vi "Test1.vi"() -> ()   [LabVIEW 2012]
uses:
  <vilib>/Rock Robotics/SystemInterfaces/DIO/FPGA_DIOPWMChannel.ctl
  <vilib>/Rock Robotics/SystemInterfaces/Typedef/FPGA_TypedefDigitalModule.ctl
  <vilib>/Rock Robotics/SystemInterfaces/DIO/FPGA_DIOChannel.ctl
  <vilib>/Rock Robotics/WPI/Encoder/WPI_EncoderType.ctl
  <vilib>/Rock Robotics/WPI/MotorControl/WPI_MotorControlOpen Talon.vi
  <vilib>/Rock Robotics/WPI/Counter/WPI_CounterDigitalInputToDigitalSource.vi
  <vilib>/addons/control/pid/pid.llb/PID (DBL).vi
  <vilib>/addons/control/pid/NI_PID_pid.lvlib
panel:
  out "Numeric":dbl
  in  "stop":bool
  out "Times run":i32
  out "Ready To Fire":bool
  in  "Shooter Speed":dbl format="%.2f"
  in  "PID gains":T1={"proportional gain (Kc)"=1.0, "integral time (Ti, min)"=0.01, "derivative time (Td, min)"=0.0} {"derivative time (Td, min)" format="%.3f"; "integral time (Ti, min)" format="%.3f"; "proportional gain (Kc)" format="%.3f"}
  in  "Maximum Encoder speed":dbl=25000.0
  in  "Shooter On":bool
  # "This is the new code for the Shooter Motors. Check and make sure that all of the controls/indecators below work and that \nit exports the data to the dashboard correctly"
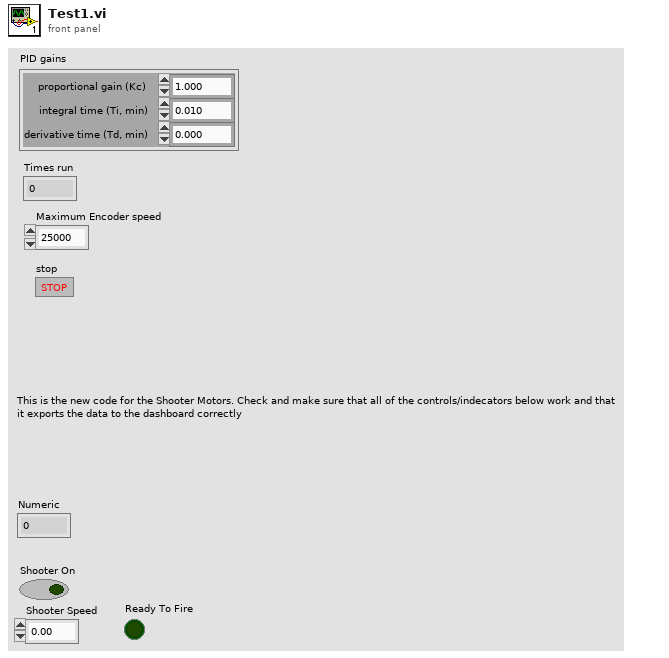
[diagram p1: front panel]
types:
  T1 = cluster{"proportional gain (Kc)":dbl, "integral time (Ti, min)":dbl, "derivative time (Td, min)":dbl}
  T2 = typedef "WPI_EncoderType.ctl" = enum16{"1x", "2x", "4x"}
  T3 = typedef "FPGA_DIOChannel.ctl" = enum8{"DIO 1", "DIO 2", "DIO 3", "DIO 4", "DIO 5", "DIO 6", "DIO 7", "DIO 8", "DIO 9", "DIO 10", "DIO 11", "DIO 12", "DIO 13", "DIO 14", "Invalid"}
  T4 = typedef "FPGA_DIOPWMChannel.ctl" = enum8{"PWM 1", "PWM 2", "PWM 3", "PWM 4", "PWM 5", "PWM 6", "PWM 7", "PWM 8", "PWM 9", "PWM 10", "Invalid"}
  T5 = typedef "FPGA_TypedefDigitalModule.ctl" = enum16{"Digital Module 1", "Digital Module 2"}
  T6 = typedef "WPI_DigitalInputDevRef.ctl" = cluster{"DevStatus":errorcluster, "DIO Channel":T3, "Digital Module":T5}
  T7 = typedef "FPGA_CounterEncoderSourceConvertionLVSourceType.ctl" = cluster{"DevStatus":errorcluster, "AnalogTriggerMode?":bool, "DigitalMode":cluster{"Digital Module":T5, "DIO Channel":T8}, "AnalogTriggerMode":cluster{"AnalogTriggerIndex":T9, "OutputType":T10}}
  T8 = typedef "FPGA_DIODigitalSourceChannel.ctl" = enum8{"DIO 1", "DIO 2", "DIO 3", "DIO 4", "DIO 5", "DIO 6", "DIO 7", "DIO 8", "DIO 9", "DIO 10", "DIO 11", "DIO 12", "DIO 13", "DIO 14", "Disabled"}
  T9 = typedef "FPGA_AnalogTriggerIndex.ctl" = enum8{"Trig 0", "Trig 1", "Trig 2", "Trig 3", "Trig 4", "Trig 5", "Trig 6", "Trig 7", "Invalid"}
  T10 = typedef "FPGA_AnalogTriggerOutType.ctl" = enum16{"InWindow", "TriggerState", "Rising", "Falling"}
  T11 = typedef "WPI_MotorControlDeviceRef.ctl" = cluster{"DeviceStatus":errorcluster, "Type":enum16{"PWM", "CAN"}, "PWM":cluster{"Digital Module":T5, "PWM Channel":T4, "DeadBand":T12}, "CAN":cluster{"Device Number":u8, "Control Mode":T13, "Semaphore":T14, "Max Vout":dbl}, "Invert":bool, "TransformRef":T15, "InvTransformRef":T15}
  T12 = typedef "WPI_PWMDeadband.ctl" = cluster{"Name":string, "maxPositivePwm":i32, "minPositivePwm":i32, "centerPwm":i32, "maxNegativePwm":i32, "minNegativePwm":i32, "angularRange":u16}
  T13 = typedef "WPI_CANJaguar_ControlMode.ctl" = enum8{"Percent VBus", "Current", "Speed", "Position", "Voltage"}
  T14 = typedef "Semaphore RefNum" = refnum<k1>
  T15 = typedef "WPI_PWMTransform_ConPane.ctl" = refnum<vi>
  T16 = typedef "WPI_EncoderDevRef.ctl" = cluster{"DevStatus":errorcluster, "EncoderIndex":T17, "CounterIndex":T18, "DistancePerCount":dbl, "Decoding Type":T2}
  T17 = typedef "FPGA_EncoderIdx.ctl" = enum8{"Enc 0", "Enc 1", "Enc 2", "Enc 3", "Invalid"}
  T18 = typedef "FPGA_CounterCtrSystemIndex.ctl" = enum8{"Ctr 0", "Ctr 1", "Ctr 2", "Ctr 3", "Ctr 4", "Ctr 5", "Ctr 6", "Ctr 7", "Invalid"}
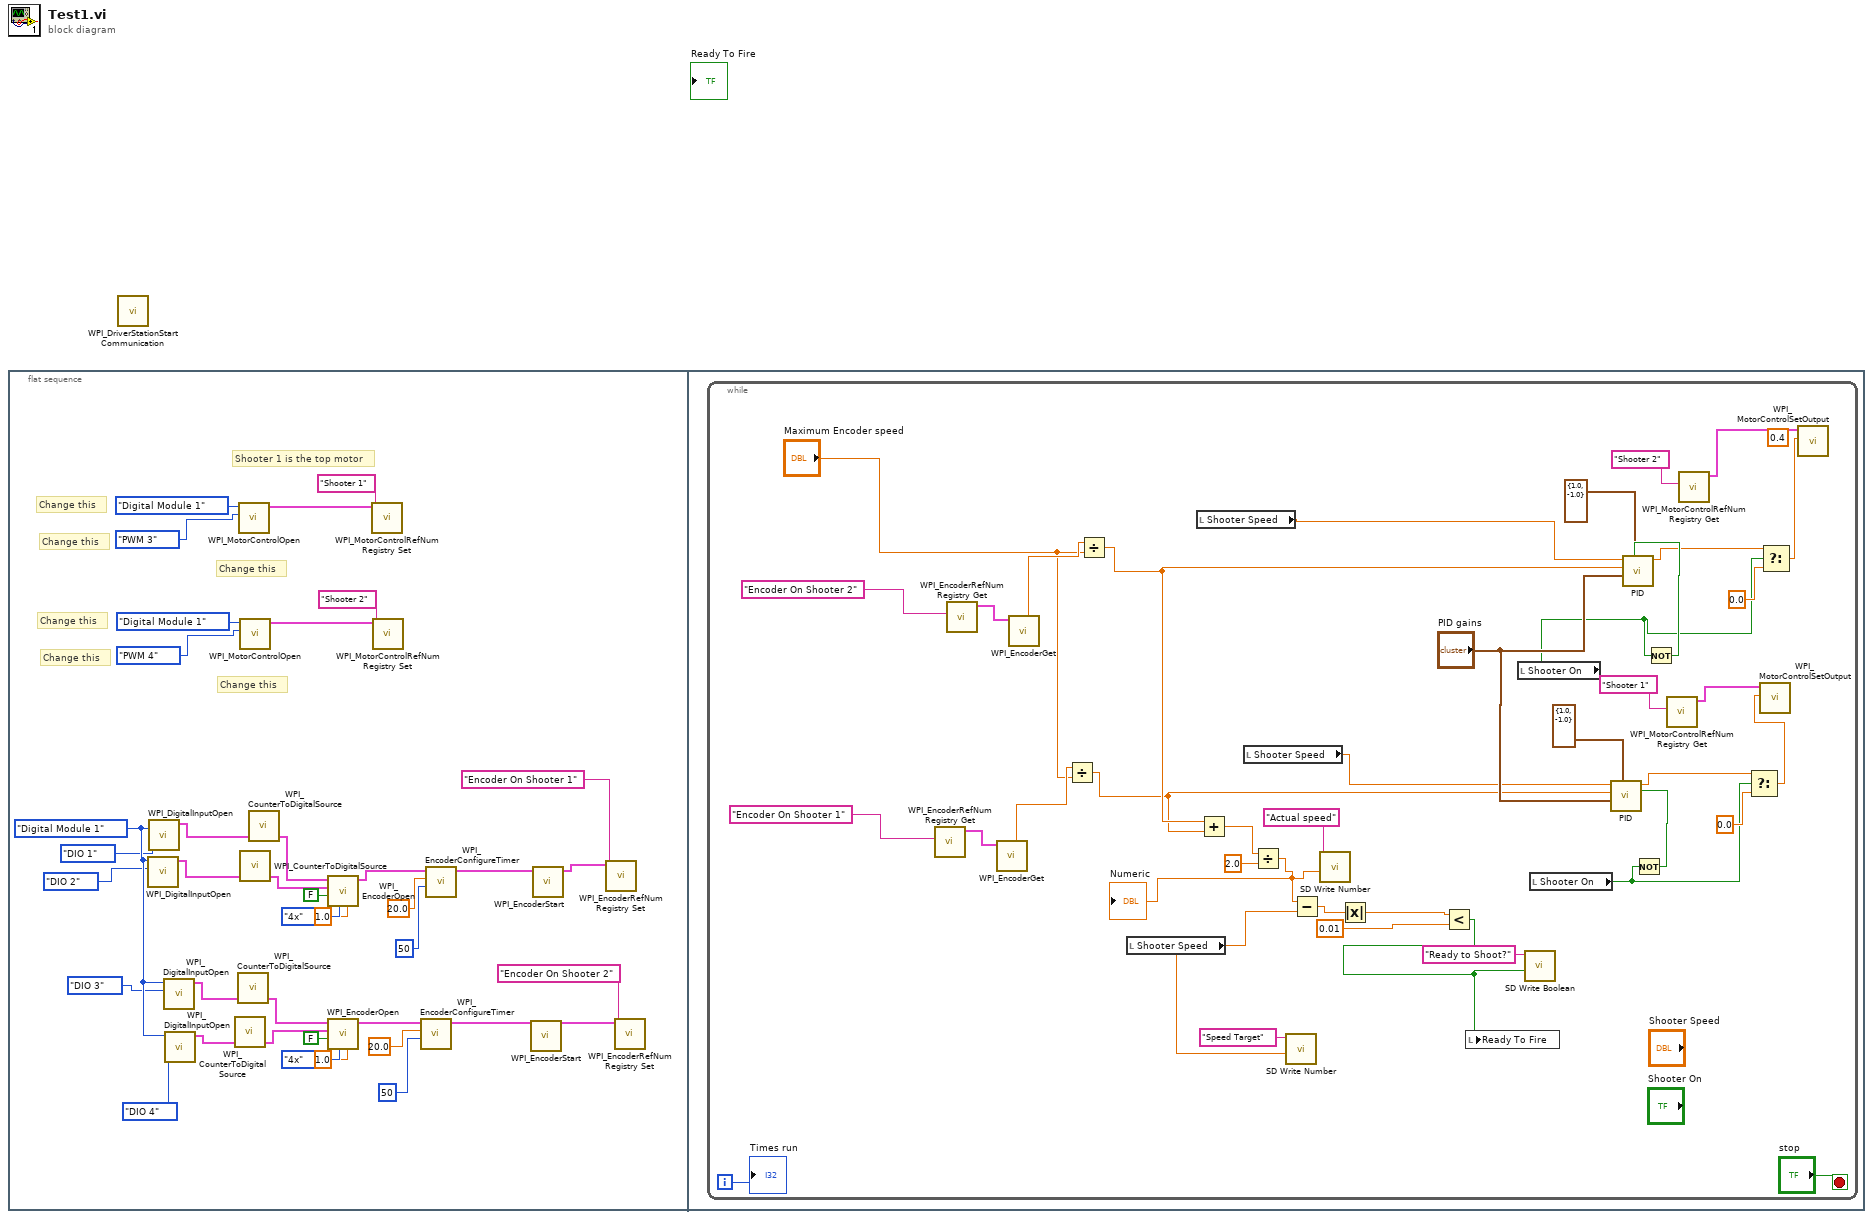
[diagram p0: block diagram]
diagram:
  n1 = flat-sequence {
    frame #0 {
      w31 = FPGA_TypedefDigitalModule."Digital Module 1" ("Digital Module (Module 1)")
      # "Shooter 1 is the top motor"
      # "Change this"
      # "Change this"
      # "Change this"
      # "Change this"
      # "Change this"
      # "Change this"
      n2 = call <vilib>:"WPI_DigitalInputOpen.vi"("DIO Channel"=FPGA_DIOChannel."DIO 2", "Digital Module (Module 1)"=w31) -> ("DigitalInputDevRef"=w24:T6)  [unwired: 8 in, 1 out]
      n3 = call <vilib>:"WPI_DigitalInputOpen.vi"("DIO Channel"=FPGA_DIOChannel."DIO 1", "Digital Module (Module 1)"=w31) -> ("DigitalInputDevRef"=w23:T6)  [unwired: 8 in, 1 out]
      n4 = call <vilib>:"WPI_DigitalInputOpen.vi"("DIO Channel"=FPGA_DIOChannel."DIO 3", "Digital Module (Module 1)"=w31) -> ("DigitalInputDevRef"=w25:T6)  [unwired: 8 in, 1 out]
      n5 = call <vilib>:"WPI_DigitalInputOpen.vi"("DIO Channel"=FPGA_DIOChannel."DIO 4", "Digital Module (Module 1)"=w31) -> ("DigitalInputDevRef"=w26:T6)  [unwired: 8 in, 1 out]
      n6 = call-poly <vilib>:"WPI_CounterToDigitalSource.vi"("DigitalInputDevRef"=w26) -> ("Digital Source"=w19:T7)  [unwired: 6 in]
      n7 = call-poly <vilib>:"WPI_CounterToDigitalSource.vi"("DigitalInputDevRef"=w25) -> ("Digital Source"=w20:T7)  [unwired: 6 in]
      n8 = call-poly <vilib>:"WPI_MotorControlOpen.vi"("PWM Channel"=FPGA_DIOPWMChannel."PWM 3", "Digital Module (Module 1)"=FPGA_TypedefDigitalModule."Digital Module 1") -> ("MotorControlDeviceRef"=w37:T11)  [unwired: 8 in, 1 out]
      n9 = call-poly <vilib>:"WPI_MotorControlOpen.vi"("PWM Channel"=FPGA_DIOPWMChannel."PWM 4", "Digital Module (Module 1)"=FPGA_TypedefDigitalModule."Digital Module 1") -> ("MotorControlDeviceRef"=w33:T11)  [unwired: 8 in, 1 out]
      n10 = call-poly <vilib>:"WPI_CounterToDigitalSource.vi"("DigitalInputDevRef"=w24) -> ("Digital Source"=w21:T7)  [unwired: 6 in]
      n11 = call-poly <vilib>:"WPI_CounterToDigitalSource.vi"("DigitalInputDevRef"=w23) -> ("Digital Source"=w22:T7)  [unwired: 6 in]
      n12 = call <vilib>:"WPI_EncoderOpen.vi"("DistancePerCount"=1.0, "Decoding Type"=WPI_EncoderType."4x", "Invert Direction (False)"=FALSE, "BSource"=w21, "ASource"=w22) -> ("EncoderDevRef"=w18:T16)  [unwired: 5 in, 1 out]
      n13 = call <vilib>:"WPI_EncoderOpen.vi"("DistancePerCount"=1.0, "Decoding Type"=WPI_EncoderType."4x", "Invert Direction (False)"=FALSE, "BSource"=w19, "ASource"=w20) -> ("EncoderDevRef"=w17:T16)  [unwired: 5 in, 1 out]
      n14 = call <vilib>:"WPI_MotorControlRefNum Registry Set.vi"("refnum name"="Shooter 1", "MotorControlDevRef"=w37) -> ()  [unwired: 8 in, 2 out]
      n15 = call <vilib>:"WPI_MotorControlRefNum Registry Set.vi"("refnum name"="Shooter 2", "MotorControlDevRef"=w33) -> ()  [unwired: 8 in, 2 out]
      n16 = call <vilib>:"WPI_EncoderConfigureTimer.vi"("Number Samples to Average"=u8 50, "Minimum Rate"=20.0, "EncoderDevRef"=w17) -> ("EncoderDevRef"=w15:T16)  [unwired: 7 in, 1 out]
      n17 = call <vilib>:"WPI_EncoderConfigureTimer.vi"("Number Samples to Average"=u8 50, "Minimum Rate"=20.0, "EncoderDevRef"=w18) -> ("EncoderDevRef"=w16:T16)  [unwired: 7 in, 1 out]
      n18 = call <vilib>:"WPI_EncoderStart.vi"("EncoderDevRef"=w15) -> ("EncoderDevRef"=w14:T16)  [unwired: 9 in, 1 out]
      n19 = call <vilib>:"WPI_EncoderStart.vi"("EncoderDevRef"=w16) -> ("EncoderDevRef"=w13:T16)  [unwired: 9 in, 1 out]
      n20 = call <vilib>:"WPI_EncoderRefNum Registry Set.vi"("refnum name"="Encoder On Shooter 1", "EncoderDevRef"=w13) -> ()  [unwired: 8 in, 2 out]
      n21 = call <vilib>:"WPI_EncoderRefNum Registry Set.vi"("refnum name"="Encoder On Shooter 2", "EncoderDevRef"=w14) -> ()  [unwired: 8 in, 2 out]
    }
    frame #1 {
      n22 = while {
        i -> [w44]
        stop <- "stop" stop-if-true
        (unwired) 0.4 ("Output")
        n23 = call <vilib>:"WPI_EncoderRefNum Registry Get.vi"("refnum name"="Encoder On Shooter 1") -> ("EncoderDevRef"=w77:T16)  [unwired: 9 in, 1 out]
        n24 = call <vilib>:"WPI_EncoderRefNum Registry Get.vi"("refnum name"="Encoder On Shooter 2") -> ("EncoderDevRef"=w68:T16)  [unwired: 9 in, 1 out]
        n25 = call <vilib>:"WPI_EncoderGet.vi"("EncoderDevRef"=w77) -> ("Rate"=w62:dbl)  [unwired: 5 in, 5 out]
        n26 = call <vilib>:"WPI_EncoderGet.vi"("EncoderDevRef"=w68) -> ("Rate"=w61:dbl)  [unwired: 5 in, 5 out]
        n27 = Divide(x=w62, y="Maximum Encoder speed") -> (x/y=w53:dbl)
        n28 = Divide(x=w61, y="Maximum Encoder speed") -> (x/y=w54:dbl)
        n29 = local read "Shooter Speed"() -> (w42:dbl)
        n30 = local read "Shooter Speed"() -> (w56:dbl)
        n31 = Add(x=w54, y=w53) -> (x+y=w52:dbl)
        n32 = local read "Shooter Speed"() -> (w57:dbl)
        n33 = Divide(x=w52, y=2.0) -> (x/y=w41:dbl)
        "Numeric" <- w41
        n34 = call <vilib>:"SD Write Number.vi"("Numeric"=w42, "Name"="Speed Target") -> ()  [unwired: 8 in, 2 out]
        n35 = Subtract(x=w41, y=w42) -> (x-y=w49:dbl)
        n36 = call <vilib>:"SD Write Number.vi"("Numeric"=w41, "Name"="Actual speed") -> ()  [unwired: 8 in, 2 out]
        n37 = Absolute Value(x=w49) -> (abs(x)=w48:dbl)
        n38 = Less?(x=w48, y=0.01) -> (x < y?=w45:bool)
        n39 = local write "Ready To Fire"(w45) -> ()
        n40 = local read "Shooter On"() -> (w59:bool)
        n41 = call <vilib>:"SD Write Boolean.vi"("Boolean"=w45, "Name"="Ready to Shoot?") -> ()  [unwired: 8 in, 2 out]
        n42 = local read "Shooter On"() -> (w58:bool)
        n43 = Not(x=w58) -> (.not. x?=w79:bool)
        n44 = call-poly <vilib>:"PID.vi"("reinitialize? (F)"=w79, "output range"=cluster{"output high":dbl, "output low":dbl} {"output high"=1.0, "output low"=-1.0}, "PID gains"="PID gains", "process variable"=w53, "setpoint"=w57) -> ("output"=w78:dbl)  [unwired: 5 in, 1 out]
        n45 = Not(x=w59) -> (.not. x?=w70:bool)
        n46 = call-poly <vilib>:"PID.vi"("reinitialize? (F)"=w70, "output range"=cluster{"output high":dbl, "output low":dbl} {"output high"=1.0, "output low"=-1.0}, "PID gains"="PID gains", "process variable"=w54, "setpoint"=w56) -> ("output"=w69:dbl)  [unwired: 5 in, 1 out]
        n47 = call <vilib>:"WPI_MotorControlRefNum Registry Get.vi"("refnum name"="Shooter 1") -> ("MotorControlDevRef"=w72:T11)  [unwired: 9 in, 1 out]
        n48 = call <vilib>:"WPI_MotorControlRefNum Registry Get.vi"("refnum name"="Shooter 2") -> ("MotorControlDevRef"=w64:T11)  [unwired: 9 in, 1 out]
        n49 = Select(t=w78, s=w58, f=0.0) -> (s? t:f=w74:dbl)
        n50 = call <vilib>:"WPI_MotorControlSetOutput.vi"("Output"=w74, "MotorControlDevRef"=w72) -> ()  [unwired: 7 in, 3 out]
        n51 = Select(t=w69, s=w59, f=0.0) -> (s? t:f=w40:dbl)
        n52 = call <vilib>:"WPI_MotorControlSetOutput.vi"("Output"=w40, "MotorControlDevRef"=w64) -> ()  [unwired: 7 in, 3 out]
        "Times run" <- w44
      }
    }
  }
  n53 = call <vilib>:"WPI_DriverStationStart Communication.vi"() -> ()  [unwired: 1 in, 11 out]
